vi "复件DAQ_DO.vi"(8 "error in":errorcluster, 11 "device in":tag="Dev1") -> (0 "error out":errorcluster)   [LabVIEW 2013]
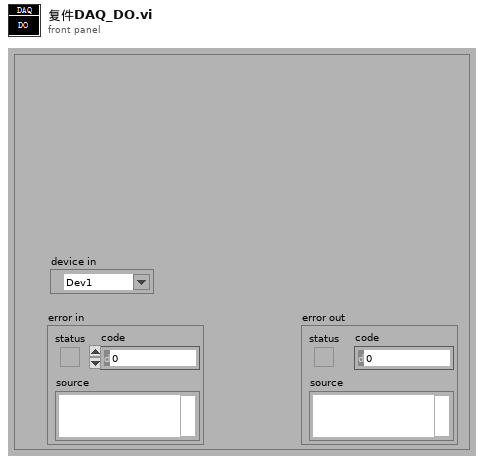
[diagram p1: front panel]
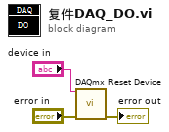
[diagram p0: block diagram]
diagram:
  n1 = call <vilib>:"DAQmx Reset Device.vi"("device in"="device in", "error in"="error in") -> ("error out"=→"error out":errorcluster)  [unwired: 13 in]
